vi "Power.vi"(10 "current waveform":waveform(dbl), 11 "voltage waveform":waveform(dbl)) -> (3 "power value":T1)   [LabVIEW 2017]
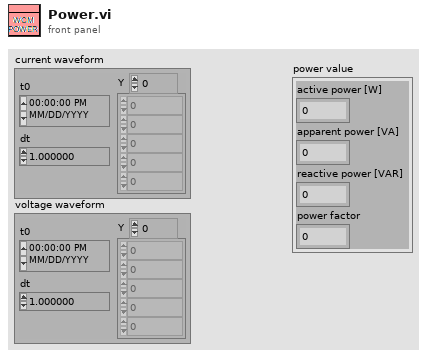
[diagram p1: front panel]
types:
  T1 = cluster{"active power [W]":dbl, "apparent power [VA]":dbl, "reactive power [VAR]":dbl, "power factor":dbl}
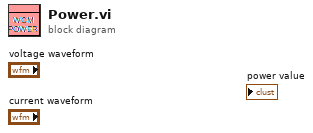
[diagram p0: block diagram]
diagram:
